vi "transition.vi"(8 "error in (no error)":errorcluster, 10 "ContextData In":refnum<class "ContextData.lvclass">, 11 "Current State":refnum<class "State.lvclass">) -> (0 "error out":errorcluster, 2 "ContextData Out":refnum<class "ContextData.lvclass">, 3 "Next State":refnum<class "State.lvclass">)   [LabVIEW 2019, in "State.lvclass"]
doc: "Invokes the transition routine of the state. Every State subclass must implement its vesion of this method. \n\nIt should contain the transition logic."
uses:
  State.lvclass
  ContextData/ContextData.lvclass
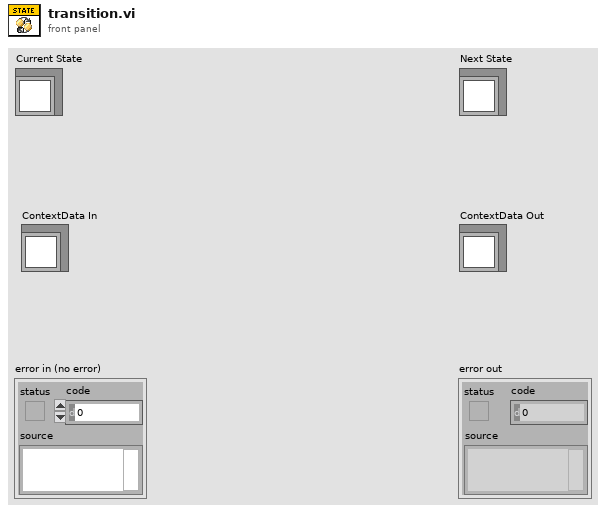
[diagram p1: front panel]
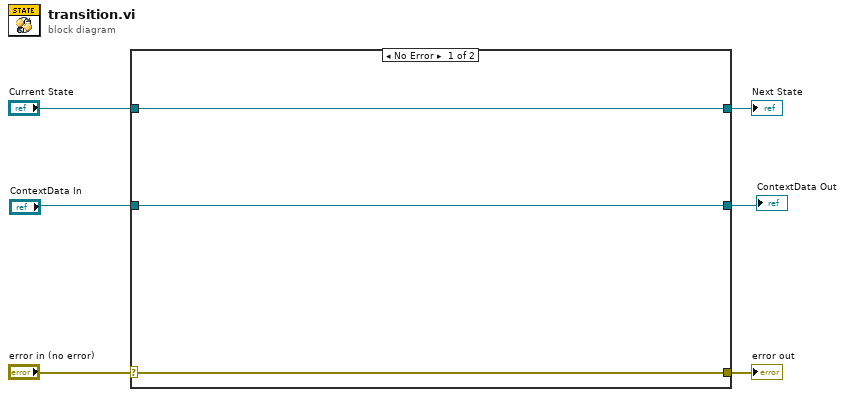
[diagram p0: block diagram]
diagram:
  n1 = case shown="No Error" "error in (no error)" {
    selector: "error in (no error)" -> [w9 w11]
    tunnel: [w9 w11] -> w5
    tunnel: [w7 w12] -> w3
    tunnel: "Current State" -> [w7 w12]
    tunnel: [w8 w10] -> w2
    tunnel: "ContextData In" -> [w8 w10]
    frame No Error {
    }
    frame Error {
      # "Wire the error cluster across even in the \"No Error\"\ncase so that warnings get propagated."
    }
  }
  "error out" <- w5
  "Next State" <- w3
  "ContextData Out" <- w2
